vi "#193_MAV_MSG_EKF_STATUS_REPORT_DECODE.vi"(11 "mavlink_payload":u8[](array[numeric])) -> (3 "EKF_STATUS_REPORT":T1)   [LabVIEW 2023]
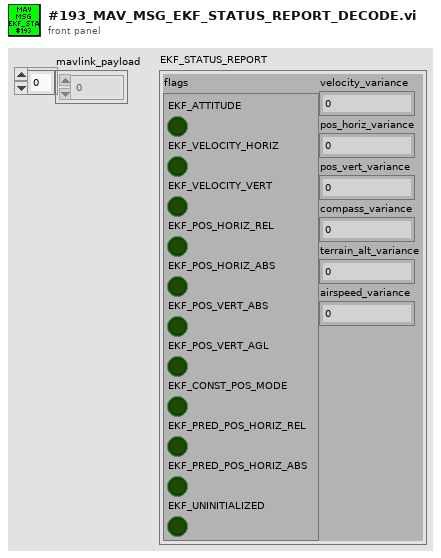
[diagram p1: front panel]
types:
  T1 = cluster{"flags":cluster{"EKF_ATTITUDE":bool, "EKF_VELOCITY_HORIZ":bool, "EKF_VELOCITY_VERT":bool, "EKF_POS_HORIZ_REL":bool, "EKF_POS_HORIZ_ABS":bool, "EKF_POS_VERT_ABS":bool, "EKF_POS_VERT_AGL":bool, "EKF_CONST_POS_MODE":bool, "EKF_PRED_POS_HORIZ_REL":bool, "EKF_PRED_POS_HORIZ_ABS":bool, "EKF_UNINITIALIZED":bool}, "velocity_variance":sgl, "pos_horiz_variance":sgl, "pos_vert_variance":sgl, "compass_variance":sgl, "terrain_alt_variance":sgl, "airspeed_variance":sgl}
  T2 = cluster{"Boolean array[0]":bool, "Boolean array[1]":bool, "Boolean array[2]":bool, "Boolean array[3]":bool, "Boolean array[4]":bool, "Boolean array[5]":bool, "Boolean array[6]":bool, "Boolean array[7]":bool, "Boolean array[8]":bool, "Boolean array[9]":bool, "Boolean array[10]":bool}
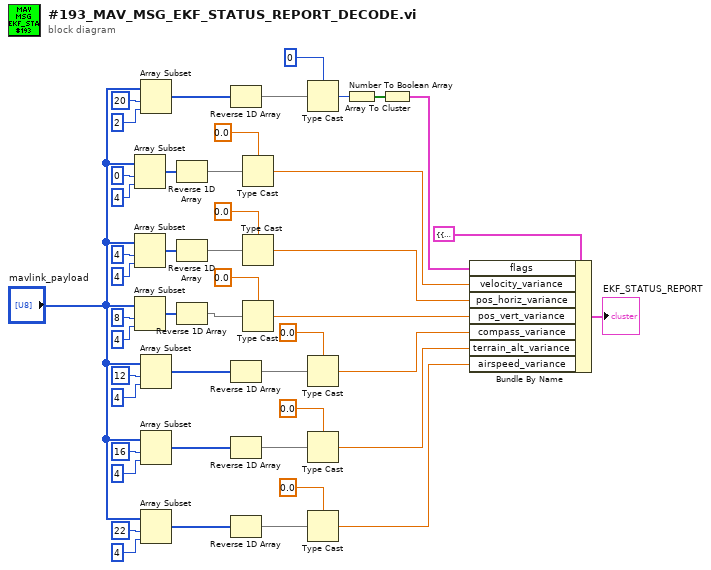
[diagram p0: block diagram]
diagram:
  n1 = Array Subset(array="mavlink_payload", index=0 ("Index"), length=4) -> (w36:u8[])
  n2 = Array Subset(array="mavlink_payload", index=4 ("Index"), length=4) -> (w30:u8[])
  n3 = Array Subset(array="mavlink_payload", index=8 ("Index"), length=4) -> (w24:u8[])
  n4 = Array Subset(array="mavlink_payload", index=20 ("Index"), length=2) -> (w45:u8[])
  n5 = Array Subset(array="mavlink_payload", index=12 ("Index"), length=4) -> (w18:u8[])
  n6 = Array Subset(array="mavlink_payload", index=16 ("Index"), length=4) -> (w12:u8[])
  n7 = Array Subset(array="mavlink_payload", index=22 ("Index"), length=4) -> (w7:u8[])
  n8 = Reverse 1D Array(array=w36) -> (reversed array=w34:u8[])
  n9 = Reverse 1D Array(array=w30) -> (reversed array=w28:u8[])
  n10 = Reverse 1D Array(array=w24) -> (reversed array=w22:u8[])
  n11 = Reverse 1D Array(array=w45) -> (reversed array=w43:u8[])
  n12 = Reverse 1D Array(array=w18) -> (reversed array=w16:u8[])
  n13 = Reverse 1D Array(array=w12) -> (reversed array=w10:u8[])
  n14 = Reverse 1D Array(array=w7) -> (reversed array=w5:u8[])
  n15 = Type Cast(type=sgl 0.0 ("Index"), x=w34) -> (*(type *) &x=w32:sgl)
  n16 = Type Cast(type=sgl 0.0 ("Index"), x=w28) -> (*(type *) &x=w26:sgl)
  n17 = Type Cast(type=sgl 0.0 ("Index"), x=w22) -> (*(type *) &x=w20:sgl)
  n18 = Type Cast(type=u16 0 ("Index"), x=w43) -> (*(type *) &x=w42:u16)
  n19 = Type Cast(type=sgl 0.0 ("Index"), x=w16) -> (*(type *) &x=w14:sgl)
  n20 = Type Cast(type=sgl 0.0 ("Index"), x=w10) -> (*(type *) &x=w2:sgl)
  n21 = Type Cast(type=sgl 0.0 ("Index"), x=w5) -> (*(type *) &x=w1:sgl)
  n22 = Number To Boolean Array(number=w42) -> (Boolean array=w47:bool[])
  n23 = Array To Cluster(array=w47) -> (cluster=w38:T2)
  n24 = Bundle By Name(cluster=T1 {"flags"={"EKF_ATTITUDE"=FALSE, "EKF_VELOCITY_HORIZ"=FALSE, "EKF_VELOCITY_VERT"=FALSE, "EKF_POS_HORIZ_REL"=FALSE, "EKF_POS_HORIZ_ABS"=FALSE, "EKF_POS_VERT_ABS"=FALSE, "EKF_POS_VERT_AGL"=FALSE, "EKF_CONST_POS_MODE"=FALSE, "EKF_PRED_POS_HORIZ_REL"=FALSE, "EKF_PRED_POS_HORIZ_ABS"=FALSE, "EKF_UNINITIALIZED"=FALSE}, "velocity_variance"=0.0, "pos_horiz_variance"=0.0, "pos_vert_variance"=0.0, "compass_variance"=0.0, "terrain_alt_variance"=0.0, "airspeed_variance"=0.0} ("EKF_STATUS_REPORT"), "flags"=w38, "velocity_variance"=w32, "pos_horiz_variance"=w26, "pos_vert_variance"=w20, "compass_variance"=w14, "terrain_alt_variance"=w2, "airspeed_variance"=w1) -> (→"EKF_STATUS_REPORT":T1)
